vi "Analytical Inverse Kinematics (6R Type 2).vi"(8 "error in (no error)":errorcluster, 10 "end effector transform":T1, 11 "6R type 2 serial arm in":refnum<class "NI_Robotics_6R Type 2 Serial Arm Class.lvclass">) -> (0 "error out":errorcluster, 1 "number of valid solutions":i32, 2 "joint positions":T1, 3 "6R type 2 serial arm out":refnum<class "NI_Robotics_6R Type 2 Serial Arm Class.lvclass">)   [LabVIEW 2017, in "NI_Robotics_6R Type 2 Serial Arm Class.lvclass"]
doc: "Returns the joint angles of a 6R, 5R, or SCARA arm given the posture of the end effector relative to the arm base. Wire data to the <B>X</B><B>_serial arm in</B> input, where <B>X</B> is the arm type, to determine the polymorphic instance to use or manually select the instance."
uses:
  <vilib>/robotics/Kinematics/Analytical/6R/Type 2/NI_Robotics_6R Type 2 Serial Arm Class.lvclass
  c:/Program Files (x86)/National Instruments/LabVIEW 2017/vi.lib/robotics/Kinematics/Robot/NI_Robotics_Serial Robot Arm.lvclass
  c:/Program Files (x86)/National Instruments/LabVIEW 2017/vi.lib/robotics/Kinematics/Analytical/Generic/NI_Robotics_Analytical Serial Arm Class.lvclass
  <vilib>/Analysis/Matrix/Datatypes/RealMatrix.ctl
  <vilib>/robotics/Kinematics/Link/NI_Robotics_Link.lvclass/NI_Robotics_Link.ctl
  <vilib>/Analysis/baseanly.llb/Real A x B.vi
  <vilib>/robotics/Kinematics/Link/Get Kinematic Parameters.vi
  <vilib>/robotics/Kinematics/Analytical/Generic/NI_Robotics_Analytical Serial Arm Class.lvclass
  <vilib>/robotics/Kinematics/Analytical/Generic/Accessors/Read alpha_n0.vi
  <vilib>/robotics/Kinematics/Robot/Get Links.vi
  <vilib>/Analysis/baseanly.llb/Real Inverse Matrix.vi
  <vilib>/robotics/Kinematics/Robot/NI_Robotics_Serial Robot Arm.lvclass
  <vilib>/Analysis/NI_AALBase.lvlib
  <vilib>/robotics/Kinematics/NI_Kinematics.lvlib
  <vilib>/Analysis/Matrix/NI_Matrix.lvlib
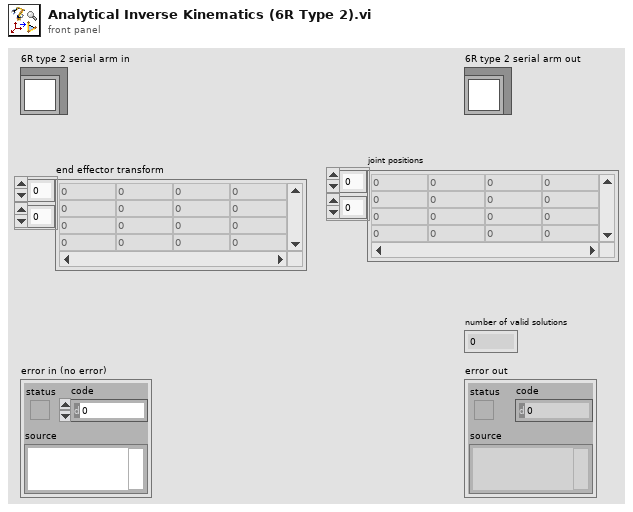
[diagram p1: front panel]
types:
  T1 = typedef "NI_Matrix.lvlib/RealMatrix.ctl" = dbl[][]
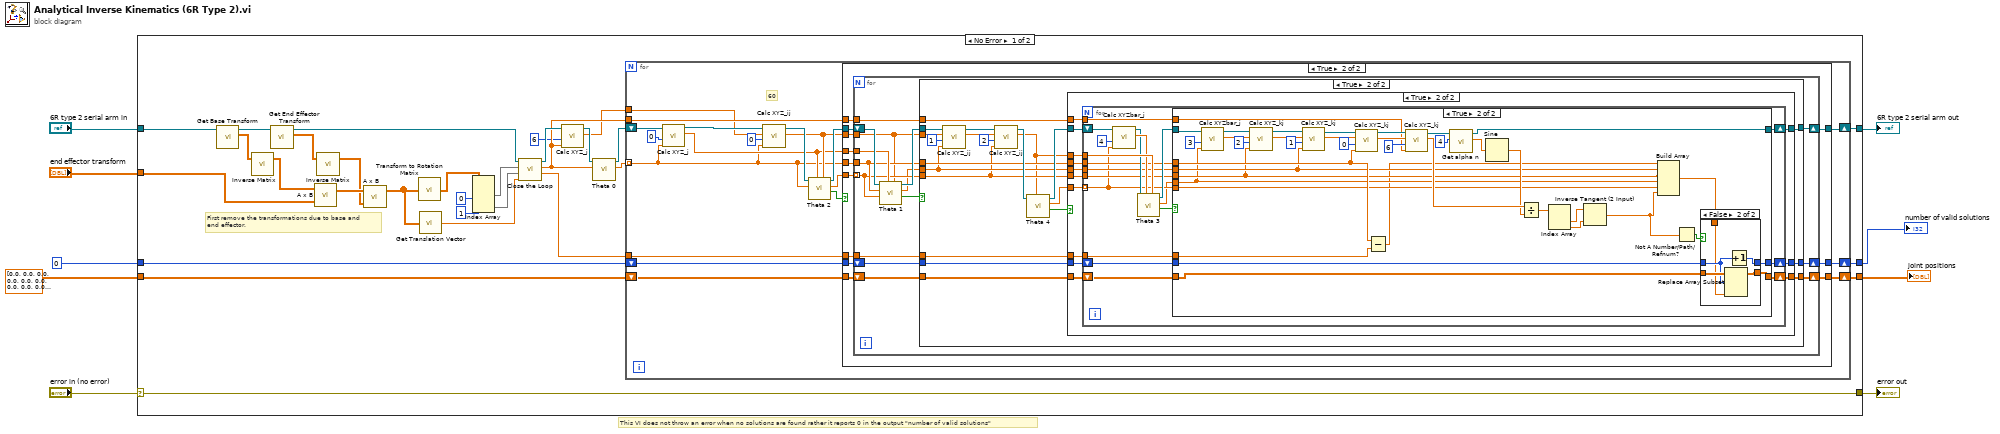
[diagram p0: block diagram]
diagram:
  # "This VI does not throw an error when no solutions are found rather it reports 0 in the output \"number of valid solutions\""
  n1 = case shown="No Error" "error in (no error)" {
    selector: "error in (no error)" -> [w39 w197]
    tunnel: [w39 w197] -> w8
    tunnel: [w21 w196] -> w6
    tunnel: "6R type 2 serial arm in" -> [w23 w196]
    tunnel: "end effector transform" -> [w24 _]
    tunnel: dbl[][] [[0.0, 0.0, 0.0, 0.0, 0.0, 0.0], [0.0, 0.0, 0.0, 0.0, 0.0, 0.0], [0.0, 0.0, 0.0, 0.0, 0.0, 0.0], [0.0, 0.0, 0.0, 0.0, 0.0, 0.0], [0.0, 0.0, 0.0, 0.0, 0.0, 0.0], [0.0, 0.0, 0.0, 0.0, 0.0, 0.0], [0.0, 0.0, 0.0, 0.0, 0.0, 0.0], [0.0, 0.0, 0.0, 0.0, 0.0, 0.0]] ("Solutions") -> [w18 _]
    tunnel: 0 -> [w19 _]
    tunnel: [w16 _] -> w2
    tunnel: [w15 _] -> w1
    frame No Error {
      # "First remove the transformations due to base and\nend effector."
      n2 = call <vilib>:"Get Base Transform.vi"("serial arm in"=w23) -> ("base transform"=w36:T1, "serial arm out"=w38:refnum<class "NI_Robotics_6R Type 2 Serial Arm Class.lvclass">)  [unwired: 8 in, 1 out]
      n3 = call-poly <vilib>:"Inverse Matrix.vi"("Input Matrix"=w36) -> ("Inverse Matrix"=w35:T1)  [unwired: 1 in, 1 out]
      n4 = call <vilib>:"Get End Effector Transform.vi"("serial arm in"=w38) -> ("end effector transform"=w37:T1, "serial arm out"=w31:refnum<class "NI_Robotics_6R Type 2 Serial Arm Class.lvclass">)  [unwired: 8 in, 1 out]
      n5 = call-poly <vilib>:"A x B.vi"("B"=w24, "A"=w35) -> ("A x B"=w34:T1)  [unwired: 1 out]
      n6 = call-poly <vilib>:"Inverse Matrix.vi"("Input Matrix"=w37) -> ("Inverse Matrix"=w33:T1)  [unwired: 1 in, 1 out]
      n7 = call-poly <vilib>:"A x B.vi"("B"=w33, "A"=w34) -> ("A x B"=w32:T1)  [unwired: 1 out]
      n8 = call <vilib>:"Transform to Rotation Matrix.vi"("transform"=w32) -> ("rotation matrix"=w27:T1)
      n9 = call <vilib>:"Get Translation Vector.vi"("transform"=w32) -> ("translation vector"=w30:dbl[])
      n10 = Index Array(array=w27, index (col) #1=0 ("disabled index (col)"), index (col) #2=1 ("index (col)")) -> (element #1=w25:dbl[], element #2=w26:dbl[])  [unwired: 2 in]
      n11 = call <vilib>:"Close the Loop.vi"("P_toolf"=w30, "S_n-1f"=w26, "a_(n-1)nf"=w25, "Analytical Serial Arm Class in"=w31) -> ("gamma_0"=w20:dbl, "theta_n"=w12:dbl, "Analytical Serial Arm Class out"=w14:refnum<class "NI_Robotics_6R Type 2 Serial Arm Class.lvclass">)  [unwired: 5 in]
      n12 = call <vilib>:"Calc XYZ_j.vi"("theta_j"=w12, "j"=6, "Analytical Serial Arm Class in"=w14) -> ("XYZ_j"=w10:dbl[], "Analytical Serial Arm Class out"=w13:refnum<class "NI_Robotics_6R Type 2 Serial Arm Class.lvclass">)  [unwired: 7 in]
      n13 = call <vilib>:"Theta 0.vi"("theta_6"=w12, "6R Type 2 Serial Arm Class in"=w13) -> ("theta_0 array"=w17:dbl[], "6R Type 2 Serial Arm Class out"=w22:refnum<class "NI_Robotics_6R Type 2 Serial Arm Class.lvclass">)  [unwired: 8 in]
      n14 = for {
        tunnel: w17 -> [w40] mode=indexing
        tunnel: w12 -> [w47]
        shift-right: [w52] -> w21
        shift-left: w22 -> [w58]
        tunnel: w20 -> [w48]
        shift-right: [w43] -> w15
        shift-left: w18 -> [w45]
        shift-right: [w44] -> w16
        shift-left: w19 -> [w46]
        tunnel: w10 -> [w41]
        # "60"
        n15 = call <vilib>:"Calc XYZ_j.vi"("theta_j"=w40, "j"=0, "Analytical Serial Arm Class in"=w58) -> ("XYZ_j"=w49:dbl[], "Analytical Serial Arm Class out"=w42:refnum<class "NI_Robotics_6R Type 2 Serial Arm Class.lvclass">)  [unwired: 7 in]
        n16 = call <vilib>:"Calc XYZ_ij.vi"("theta_j"=w40, "j"=0, "XYZ_i"=w41, "Analytical Serial Arm Class in"=w42) -> ("XYZ_ij"=w50:dbl[], "Analytical Serial Arm Class out"=w55:refnum<class "NI_Robotics_6R Type 2 Serial Arm Class.lvclass">)  [unwired: 5 in, 1 out]
        n17 = call <vilib>:"Theta 2.vi"("XYZ_60"=w50, "XYZ_0"=w49, "theta_0"=w40, "6R Type 2 Serial Arm Class in"=w55) -> ("Valid"=w54:bool, "theta_2 array"=w51:dbl[], "6R Type 2 Serial Arm Class out"=w53:refnum<class "NI_Robotics_6R Type 2 Serial Arm Class.lvclass">)  [unwired: 5 in]
        n18 = case shown="True" w54 {
          tunnel: w40 -> [_ w70]
          tunnel: w53 -> [w61 w73]
          tunnel: [w61 w72] -> w52
          tunnel: w51 -> [_ w71]
          tunnel: w50 -> [_ w69]
          tunnel: w49 -> [_ w68]
          tunnel: w48 -> [_ w67]
          tunnel: w47 -> [_ w66]
          tunnel: w46 -> [w60 w65]
          tunnel: w45 -> [w59 w64]
          tunnel: [w60 w63] -> w44
          tunnel: [w59 w62] -> w43
          frame False {
          }
          frame True {
            n19 = for {
              shift-right: [w81] -> w72
              shift-left: w73 -> [w88]
              tunnel: w71 -> [w83] mode=indexing
              tunnel: w70 -> [w84]
              tunnel: w69 -> [w80]
              tunnel: w68 -> [w87]
              tunnel: w67 -> [w79]
              tunnel: w66 -> [w78]
              shift-right: [w74] -> w62
              shift-left: w64 -> [w76]
              shift-right: [w75] -> w63
              shift-left: w65 -> [w77]
              n20 = call <vilib>:"Theta 1.vi"("XYZ_60"=w80, "XYZ_0"=w87, "theta_2"=w83, "theta_0"=w84, "6R Type 2 Serial Arm Class in"=w88) -> ("Valid"=w85:bool, "theta1"=w82:dbl, "6R Type 2 Serial Arm Class out"=w86:refnum<class "NI_Robotics_6R Type 2 Serial Arm Class.lvclass">)  [unwired: 4 in]
              n21 = case shown="True" w85 {
                tunnel: w86 -> [w91 w112]
                tunnel: w84 -> [_ w102]
                tunnel: w83 -> [_ w100]
                tunnel: w82 -> [_ w101]
                tunnel: [w91 w104] -> w81
                tunnel: w80 -> [_ w111]
                tunnel: w79 -> [_ w95]
                tunnel: w78 -> [_ w97]
                tunnel: w77 -> [w90 w94]
                tunnel: w76 -> [w89 w96]
                tunnel: [w90 w93] -> w75
                tunnel: [w89 w92] -> w74
                frame False {
                }
                frame True {
                  n22 = call <vilib>:"Calc XYZ_ij.vi"("theta_j"=w101, "j"=1, "XYZ_i"=w111, "Analytical Serial Arm Class in"=w112) -> ("XYZ_ij"=w108:dbl[], "Analytical Serial Arm Class out"=w109:refnum<class "NI_Robotics_6R Type 2 Serial Arm Class.lvclass">)  [unwired: 5 in, 1 out]
                  n23 = call <vilib>:"Calc XYZ_ij.vi"("theta_j"=w100, "j"=2, "XYZ_i"=w108, "Analytical Serial Arm Class in"=w109) -> ("XYZ_ij"=w98:dbl[], "Analytical Serial Arm Class out"=w106:refnum<class "NI_Robotics_6R Type 2 Serial Arm Class.lvclass">)  [unwired: 5 in, 1 out]
                  n24 = call <vilib>:"Theta 4.vi"("XYZ_6012"=w98, "6R Type 2 Serial Arm Class in"=w106) -> ("Valid"=w103:bool, "theta_4 array"=w99:dbl[], "6R Type 2 Serial Arm Class out"=w105:refnum<class "NI_Robotics_6R Type 2 Serial Arm Class.lvclass">)  [unwired: 7 in]
                  n25 = case shown="True" w103 {
                    tunnel: w105 -> [w115 w128]
                    tunnel: [w115 w127] -> w104
                    tunnel: w102 -> [_ w125]
                    tunnel: w101 -> [_ w124]
                    tunnel: w100 -> [_ w123]
                    tunnel: w99 -> [_ w126]
                    tunnel: w98 -> [_ w122]
                    tunnel: w97 -> [_ w121]
                    tunnel: w96 -> [w113 w120]
                    tunnel: w95 -> [_ w119]
                    tunnel: w94 -> [w114 w118]
                    tunnel: [w114 w117] -> w93
                    tunnel: [w113 w116] -> w92
                    frame False {
                    }
                    frame True {
                      n26 = for {
                        shift-right: [w140] -> w127
                        shift-left: w128 -> [w147]
                        tunnel: w126 -> [w136] mode=indexing
                        tunnel: w125 -> [w139]
                        tunnel: w124 -> [w138]
                        tunnel: w123 -> [w137]
                        tunnel: w122 -> [w146]
                        tunnel: w121 -> [w134]
                        tunnel: w119 -> [w132]
                        shift-right: [w130] -> w116
                        shift-left: w120 -> [w133]
                        shift-right: [w129] -> w117
                        shift-left: w118 -> [w131]
                        n27 = call <vilib>:"Calc XYZbar_j.vi"("theta_j"=w136, "j"=4, "Analytical Serial Arm Class in"=w147) -> ("XYZbar_j"=w145:dbl[], "Analytical Serial Arm Class out"=w143:refnum<class "NI_Robotics_6R Type 2 Serial Arm Class.lvclass">)  [unwired: 7 in]
                        n28 = call <vilib>:"Theta 3.vi"("XYZ_6012"=w146, "XYZbar_4"=w145, "6R Type 2 Serial Arm Class in"=w143) -> ("Valid"=w142:bool, "theta_3"=w135:dbl, "6R Type 2 Serial Arm Class out"=w141:refnum<class "NI_Robotics_6R Type 2 Serial Arm Class.lvclass">)  [unwired: 6 in]
                        n29 = case shown="True" w142 {
                          tunnel: w141 -> [w150 w188]
                          tunnel: [w150 w151] -> w140
                          tunnel: w139 -> [_ w165]
                          tunnel: w138 -> [_ w163]
                          tunnel: w137 -> [_ w162]
                          tunnel: w136 -> [_ w160]
                          tunnel: w135 -> [_ w161]
                          tunnel: w134 -> [_ w174]
                          tunnel: w133 -> [w148 w154]
                          tunnel: w132 -> [_ w164]
                          tunnel: w131 -> [w149 w155]
                          tunnel: [w148 w153] -> w130
                          tunnel: [w149 w152] -> w129
                          frame False {
                          }
                          frame True {
                            n30 = call <vilib>:"Calc XYZbar_j.vi"("theta_j"=w161, "j"=3, "Analytical Serial Arm Class in"=w188) -> ("XYZbar_j"=w185:dbl[], "Analytical Serial Arm Class out"=w186:refnum<class "NI_Robotics_6R Type 2 Serial Arm Class.lvclass">)  [unwired: 7 in]
                            n31 = call <vilib>:"Calc XYZ_kj.vi"("theta_j"=w162, "j"=2, "XYZbar_k"=w185, "Analytical Serial Arm Class in"=w186) -> ("XYZ_ij"=w182:dbl[], "Analytical Serial Arm Class out"=w183:refnum<class "NI_Robotics_6R Type 2 Serial Arm Class.lvclass">)  [unwired: 5 in, 1 out]
                            n32 = call <vilib>:"Calc XYZ_kj.vi"("theta_j"=w163, "j"=1, "XYZbar_k"=w182, "Analytical Serial Arm Class in"=w183) -> ("XYZ_ij"=w179:dbl[], "Analytical Serial Arm Class out"=w180:refnum<class "NI_Robotics_6R Type 2 Serial Arm Class.lvclass">)  [unwired: 5 in, 1 out]
                            n33 = call <vilib>:"Calc XYZ_kj.vi"("theta_j"=w165, "j"=0, "XYZbar_k"=w179, "Analytical Serial Arm Class in"=w180) -> ("XYZ_ij"=w175:dbl[], "Analytical Serial Arm Class out"=w177:refnum<class "NI_Robotics_6R Type 2 Serial Arm Class.lvclass">)  [unwired: 5 in, 1 out]
                            n34 = Subtract(x=w165, y=w164) -> (x-y=w159:dbl)
                            n35 = call <vilib>:"Calc XYZ_kj.vi"("theta_j"=w174, "j"=6, "XYZbar_k"=w175, "Analytical Serial Arm Class in"=w177) -> ("XYZ_ij"=w170:dbl[], "Analytical Serial Arm Class out"=w173:refnum<class "NI_Robotics_6R Type 2 Serial Arm Class.lvclass">)  [unwired: 5 in, 1 out]
                            n36 = call <vilib>:"Get alpha n.vi"("n"=4, "Analytical Serial Arm Class in"=w173) -> ("alpha n"=w171:dbl, "Analytical Serial Arm Class out"=w151:refnum<class "NI_Robotics_6R Type 2 Serial Arm Class.lvclass">)  [unwired: 8 in]
                            n37 = Sine(x=w171) -> (sin(x)=w169:dbl)
                            n38 = Divide(x=w170, y=w169) -> (x/y=w168:dbl[])
                            n39 = Index Array(array=w168) -> (element #1=w167:dbl, element #2=w166:dbl)  [unwired: 2 in]
                            n40 = Inverse Tangent (2 Input)(1:w166, 2:w167) -> (0:w156:dbl)
                            n41 = Build Array(w159, w163, w162, w161, w160, w156) -> (w157:dbl[])
                            n42 = Not A Number/Path/Refnum?(number/path/refnum=w156) -> (NaN/Path/Refnum?=w158:bool)
                            n43 = case shown="False" w158 {
                              tunnel: w154 -> [w189 w195]
                              tunnel: [w189 w194] -> w153
                              tunnel: w155 -> [w190 w193]
                              tunnel: [w190 w192] -> w152
                              tunnel: w157 -> [_ w191]
                              frame True {
                              }
                              frame False {
                                n44 = Replace Array Subset(array=w195, new element=w191, index (row)=w193) -> (w194:dbl[][])  [unwired: 1 in]
                                n45 = Increment(x=w193) -> (x+1=w192:i32)
                              }
                            }
                          }
                        }
                      }
                    }
                  }
                }
              }
            }
          }
        }
      }
    }
    frame Error {
    }
  }
  "error out" <- w8
  "6R type 2 serial arm out" <- w6
  "joint positions" <- w1
  "number of valid solutions" <- w2
